vi "Read Device Information.vi"(8 "error in (no error)":errorcluster, 11 "Lotis in":refnum<class "PL Lotis TII LS.lvclass">) -> (0 "error out":errorcluster, 2 "information":T1 {"optical channels" items=["no", "single", "double", "double with ns delays"]; "cooling system" items=["no", "single", "double", "internal"]; "laser system" items=["single lamp", "double lamp", "long pulse", "double lamp PICO", "single lamp with delay", "extended synchronization"]}, 3 "Lotis out":refnum<class "PL Lotis TII LS.lvclass">)   [LabVIEW 2015, in "PL Lotis TII LS.lvclass"]
doc: "Reads device information."
uses:
  PL Lotis TII LS.lvclass
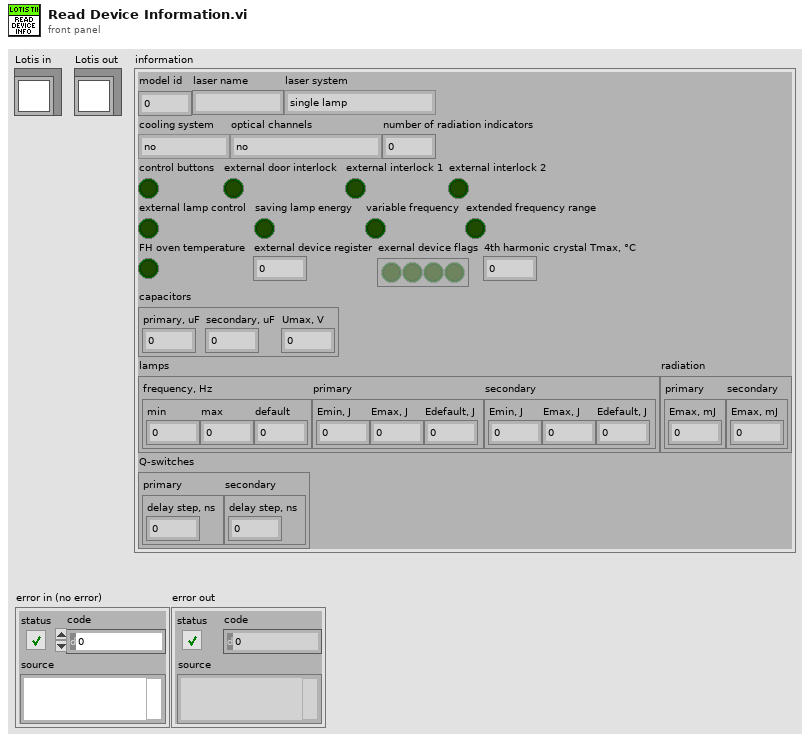
[diagram p1: front panel]
types:
  T1 = cluster{"model id":u16, "laser name":string, "laser system":u16, "optical channels":u16, "number of radiation indicators":u16, "cooling system":u16, "control buttons":bool, "external door interlock":bool, "external interlock 1":bool, "external interlock 2":bool, "external lamp control":bool, "saving lamp energy":bool, "variable frequency":bool, "extended frequency range":bool, "FH oven temperature":bool, "external device register":u8, "exernal device flags":bool[], "4th harmonic crystal Tmax, °C":u32, "capacitors":cluster{"primary, uF":u32, "secondary, uF":u32, "Umax, V":u32}, "lamps":cluster{"frequency, Hz":cluster{"min":u32, "max":u32, "default":u32}, "primary":cluster{"Emin, J":u32, "Emax, J":u32, "Edefault, J":u32}, "secondary":cluster{"Emin, J":u32, "Emax, J":u32, "Edefault, J":u32}}, "radiation":cluster{"primary":cluster{"Emax, mJ":u32}, "secondary":cluster{"Emax, mJ":u32}}, "Q-switches":cluster{"primary":cluster{"delay step, ns":u32}, "secondary":cluster{"delay step, ns":u32}}}
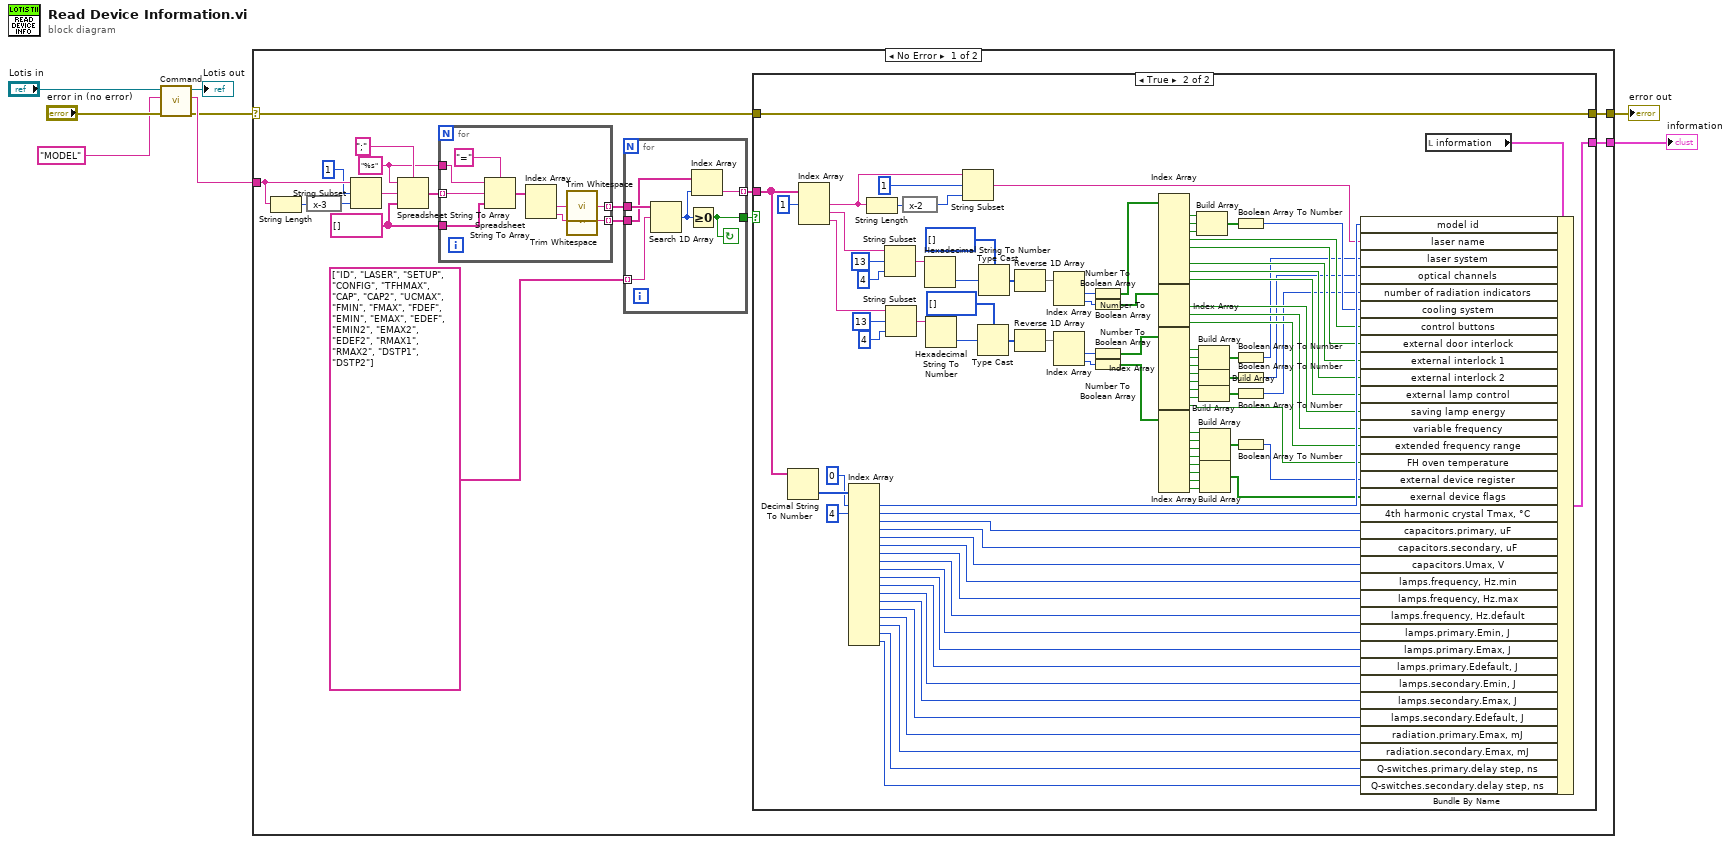
[diagram p0: block diagram]
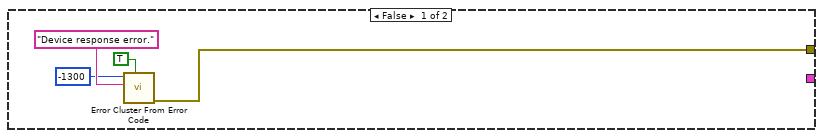
[diagram p2: hidden frame]
diagram:
  n1 = call "Command.vi"("error in (no error)"="error in (no error)", "command"="MODEL", "Lotis in"="Lotis in") -> ("error out"=w3:errorcluster, "response data"=w4:string, "Lotis out"=→"Lotis out":refnum<class "PL Lotis TII LS.lvclass">)  [unwired: 6 in]
  n2 = case shown="No Error" w3 {
    selector: w3 -> [w14 w138]
    tunnel: w4 -> [w25 _]
    tunnel: [w13 w138] -> w2
    tunnel: [w9 _] -> w1
    frame No Error {
      w18 = "%s" ("format string")
      w17 = string[] [] ("array type (2D Dbl)")
      n3 = String Length(string=w25) -> (length=w23:i32)
      n4 = expression code="x-3"(w23) -> (w22:i32)
      n5 = String Subset(string=w25, offset (0)=1, length (rest)=w22) -> (substring=w21:string)
      n6 = Spreadsheet String To Array(delimiter (Tab)=";", format string=w18, spreadsheet string=w21, array type (2D Dbl)=w17) -> (array=w19:string[])
      n7 = for {
        tunnel: w19 -> [w134] mode=indexing
        tunnel: w18 -> [w137]
        tunnel: w17 -> [w135]
        tunnel: [w130] -> w16 mode=indexing
        tunnel: [w129] -> w11 mode=indexing
        n8 = Spreadsheet String To Array(delimiter (Tab)="=", format string=w137, spreadsheet string=w134, array type (2D Dbl)=w135) -> (array=w133:string[])
        n9 = Index Array(array=w133) -> (element #1=w132:string, element #2=w131:string)  [unwired: 2 in]
        n10 = call <vilib>:"Trim Whitespace.vi"("string"=w132) -> ("trimmed string"=w130:string)  [unwired: 1 in]
        n11 = call <vilib>:"Trim Whitespace.vi"("string"=w131) -> ("trimmed string"=w129:string)  [unwired: 1 in]
      }
      n12 = for {
        tunnel: w16 -> [w128]
        tunnel: string[] ["ID", "LASER", "SETUP", "CONFIG", "TFHMAX", "CAP", "CAP2", "UCMAX", "FMIN", "FMAX", "FDEF", "EMIN", "EMAX", "EDEF", "EMIN2", "EMAX2", "EDEF2", "RMAX1", "RMAX2", "DSTP1", "DSTP2"] -> [w127] mode=indexing
        tunnel: [w126] -> w12
        tunnel: w11 -> [w125]
        tunnel: [w123] -> w10 mode=indexing
        stop <- w126 continue-if-true
        n13 = Search 1D Array(1D array=w128, element=w127) -> (index of element=w124:i32)  [unwired: 1 in]
        n14 = Greater Or Equal To 0?(x=w124) -> (x >= 0?=w126:bool)
        n15 = Index Array(array=w125, index=w124) -> (element=w123:string)
      }
      n16 = case shown="True" w12 {
        tunnel: w14 -> [_ w122]
        tunnel: [w26 w122] -> w13
        tunnel: w10 -> [_ w115]
        tunnel: [_ w120] -> w9
        frame False {
          n17 = call <vilib>:"Error Cluster From Error Code.vi"("show call chain? (False)"=TRUE, "error message (\"\")"="Device response error." ("format string"), "error code (0)"=-1300) -> ("error out"=w26:errorcluster)  [unwired: 6 in]
        }
        frame True {
          n18 = Decimal String To Number(string=w115) -> (number=w114:i32[])  [unwired: 2 in, 1 out]
          n19 = Index Array(array=w115, index #1=1 ("index")) -> (element #1=w30:string, element #2=w87:string, element #3=w81:string)  [unwired: 2 in]
          n20 = Index Array(array=w114, index #1=0 ("index"), index #2=4 ("index")) -> (element #1=w95:i32, element #2=w113:i32, element #3=w112:i32, element #4=w111:i32, element #5=w110:i32, element #6=w109:i32, element #7=w108:i32, element #8=w107:i32, element #9=w106:i32, element #10=w105:i32, element #11=w104:i32, element #12=w103:i32, element #13=w102:i32, element #14=w101:i32, element #15=w100:i32, element #16=w99:i32, element #17=w98:i32, element #18=w97:i32)  [unwired: 16 in]
          n21 = String Length(string=w30) -> (length=w118:i32)
          n22 = String Subset(string=w87, offset (0)=13, length (rest)=4 ("length (rest)")) -> (substring=w91:string)
          n23 = String Subset(string=w81, offset (0)=13, length (rest)=4 ("length (rest)")) -> (substring=w83:string)
          n24 = expression code="x-2"(w118) -> (w117:i32)
          n25 = Hexadecimal String To Number(string=w91) -> (number=w90:u32)  [unwired: 2 in, 1 out]
          n26 = Hexadecimal String To Number(string=w83) -> (number=w84:u32)  [unwired: 2 in, 1 out]
          n27 = String Subset(string=w30, offset (0)=1, length (rest)=w117) -> (substring=w93:string)
          n28 = Type Cast(type=u8[] [], x=w84) -> (*(type *) &x=w79:u8[])
          n29 = Type Cast(type=u8[] [], x=w90) -> (*(type *) &x=w80:u8[])
          n30 = Reverse 1D Array(array=w80) -> (reversed array=w78:u8[])
          n31 = Reverse 1D Array(array=w79) -> (reversed array=w77:u8[])
          n32 = Index Array(array=w78) -> (element #1=w76:u8, element #2=w73:u8)  [unwired: 2 in]
          n33 = Index Array(array=w77) -> (element #1=w75:u8, element #2=w74:u8)  [unwired: 2 in]
          n34 = Number To Boolean Array(number=w76) -> (Boolean array=w71:bool[])
          n35 = Number To Boolean Array(number=w73) -> (Boolean array=w65:bool[])
          n36 = Number To Boolean Array(number=w75) -> (Boolean array=w57:bool[])
          n37 = Number To Boolean Array(number=w74) -> (Boolean array=w56:bool[])
          n38 = Index Array(array=w71) -> (element #1=w61:bool, element #2=w59:bool, element #3=w60:bool, element #4=w70:bool, element #5=w69:bool, element #7=w68:bool, element #8=w67:bool, element #9=w66:bool)  [unwired: 9 in, 1 out]
          n39 = Index Array(array=w65) -> (element #1=w64:bool, element #2=w63:bool, element #3=w62:bool)  [unwired: 3 in]
          n40 = Index Array(array=w57) -> (element #1=w55:bool, element #2=w54:bool, element #3=w53:bool, element #4=w52:bool, element #5=w50:bool, element #6=w51:bool, element #7=w49:bool, element #8=w33:bool)  [unwired: 8 in]
          n41 = Index Array(array=w56) -> (element #1=w48:bool, element #2=w47:bool, element #3=w46:bool, element #4=w45:bool, element #5=w44:bool, element #6=w43:bool, element #7=w42:bool, element #8=w41:bool)  [unwired: 8 in]
          n42 = Build Array(w61, w59, w60) -> (w58:bool[])
          n43 = Build Array(w55, w54, w53) -> (w40:bool[])
          n44 = Build Array(w52, w50) -> (w39:bool[])
          n45 = Build Array(w51, w49) -> (w38:bool[])
          n46 = Build Array(w48, w47, w46, w45) -> (w37:bool[])
          n47 = Build Array(w44, w43, w42, w41) -> (w31:bool[])
          n48 = Boolean Array To Number(Boolean array=w58) -> (number=w72:u32)
          n49 = Boolean Array To Number(Boolean array=w40) -> (number=w36:u32)
          n50 = Boolean Array To Number(Boolean array=w39) -> (number=w35:u32)
          n51 = Boolean Array To Number(Boolean array=w38) -> (number=w34:u32)
          n52 = Boolean Array To Number(Boolean array=w37) -> (number=w32:u32)
          n53 = local read "information"() -> (w121:T1)
          n54 = Bundle By Name(cluster=w121, "model id"=w95, "laser name"=w93, "laser system"=w36, "optical channels"=w35, "number of radiation indicators"=w34, "cooling system"=w72, "control buttons"=w70, "external door interlock"=w69, "external interlock 1"=w68, "external interlock 2"=w67, "external lamp control"=w66, "saving lamp energy"=w64, "variable frequency"=w63, "extended frequency range"=w62, "FH oven temperature"=w33, "external device register"=w32, "exernal device flags"=w31, "4th harmonic crystal Tmax, °C"=w113, "capacitors.primary, uF"=w112, "capacitors.secondary, uF"=w111, "capacitors.Umax, V"=w110, "lamps.frequency, Hz.min"=w109, "lamps.frequency, Hz.max"=w108, "lamps.frequency, Hz.default"=w107, "lamps.primary.Emin, J"=w106, "lamps.primary.Emax, J"=w105, "lamps.primary.Edefault, J"=w104, "lamps.secondary.Emin, J"=w103, "lamps.secondary.Emax, J"=w102, "lamps.secondary.Edefault, J"=w101, "radiation.primary.Emax, mJ"=w100, "radiation.secondary.Emax, mJ"=w99, "Q-switches.primary.delay step, ns"=w98, "Q-switches.secondary.delay step, ns"=w97) -> (w120:T1)
        }
      }
    }
    frame Error {
    }
  }
  "error out" <- w2
  "information" <- w1
